vi "parseCCDData.vi"(8 "error in (no error)":errorcluster, 11 "results-JSON string":string) -> (0 "error out":errorcluster, 3 "Array":dbl[][][][](array[numeric]))   [LabVIEW 2023, in "CCD.lvclass"]
uses:
  CCD.lvclass
  dbdbfdab-1b16-4349-82fb-0439317991f3.vi
  <vilib>/JDP Science/JSONtext/Next JSON Value.vi
  <vilib>/JDP Science/JSONtext/String Subset.vi
  <vilib>/JDP Science/JSONtext/Parsing/Advance past next JSON Value (inlined COPY).vi
  <vilib>/JDP Science/JSONtext/Parsing/Advance past whitespace.vi
  <vilib>/JDP Science/JSONtext/Parsing/Advance past String.vi
  <vilib>/JDP Science/JSONtext/Parsing/Advance past Number.vi
  <vilib>/JDP Science/JSONtext/Parsing/Advance past Line Ending.vi
  <vilib>/JDP Science/JSONtext/Parsing/Parse Full Path or Item Name.vi
  <vilib>/JDP Science/JSONtext/Parsing/Advance past Array.vi
  <vilib>/JDP Science/JSONtext/Parsing/Advance past Object.vi
  <vilib>/JDP Science/JSONtext/support/Error Cluster From Code.vi
  <vilib>/JDP Science/JSONtext/Offset/Find Item Locations by Path.vi
  <vilib>/JDP Science/JSONtext/JSON text to Variant.vi
  <vilib>/JDP Science/JSONtext/LVClass Serializer/JSONtext LVClass Serializer.lvclass
  <vilib>/JDP Science/JSONtext/JSONtext.lvlib
  xyData.ctl
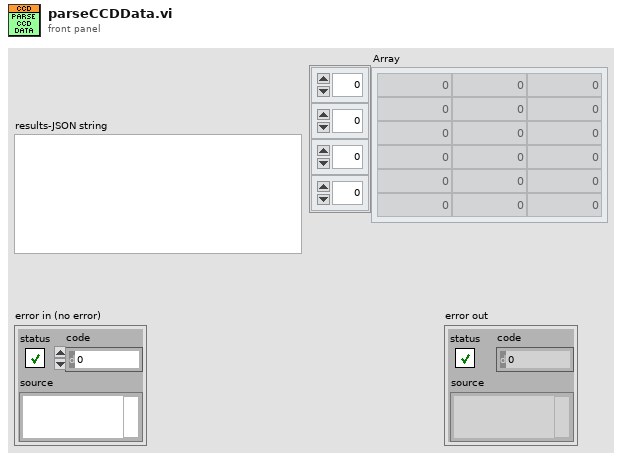
[diagram p1: front panel]
types:
  T1 = typedef "CCD.lvclass/xyData.ctl" = cluster{"xyData":dbl[][]}
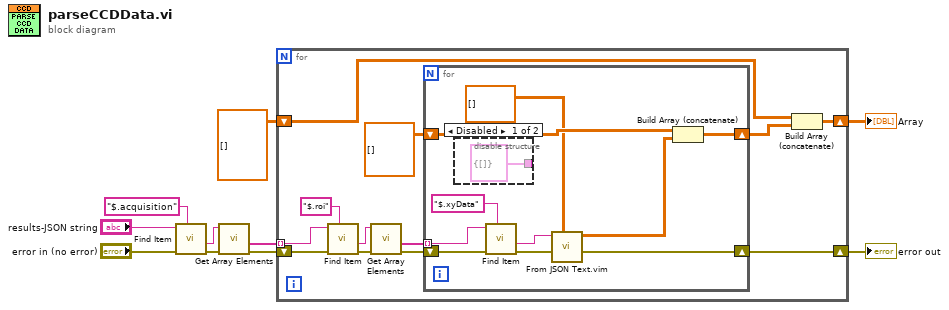
[diagram p0: block diagram]
diagram:
  n1 = call <vilib>:"Find Item.vi"("$Path or Item Name"="$.acquisition", "error in (no error)"="error in (no error)", "JSON"="results-JSON string") -> ("error out"=w7:errorcluster, "<JSON>"=w6:string)  [unwired: 5 in, 2 out]
  n2 = call <vilib>:"Get Array Elements.vi"("error in (no error)"=w7, "JSON"=w6) -> ("error out"=w10:errorcluster, "<JSON>"=w9:string[])  [unwired: 7 in, 1 out]
  n3 = for {
    tunnel: w9 -> [w16] mode=indexing
    shift-right: [w17] -> w5
    shift-left: w10 -> [w19]
    shift-right: [w13] -> w1
    shift-left: dbl[][][][] [] -> [w12]
    n4 = call <vilib>:"Find Item.vi"("$Path or Item Name"="$.roi", "error in (no error)"=w19, "JSON"=w16) -> ("error out"=w21:errorcluster, "<JSON>"=w20:string)  [unwired: 5 in, 2 out]
    n5 = call <vilib>:"Get Array Elements.vi"("error in (no error)"=w21, "JSON"=w20) -> ("error out"=w18:errorcluster, "<JSON>"=w15:string[])  [unwired: 7 in, 1 out]
    n6 = for {
      shift-right: [w28] -> w17
      shift-left: w18 -> [w30]
      tunnel: w15 -> [w31] mode=indexing
      shift-right: [w27] -> w14
      shift-left: dbl[][][] [] -> [w26]
      n7 = disable-structure shown="Disabled" {
        disable-tunnel: [T1 {"xyData"=[]} ("xyData") _] -> _
        frame Disabled {
        }
        frame Enabled {
        }
      }
      n8 = call <vilib>:"Find Item.vi"("$Path or Item Name"="$.xyData", "error in (no error)"=w30, "JSON"=w31) -> ("error out"=w29:errorcluster, "<JSON>"=w25:string)  [unwired: 5 in, 2 out]
      n9 = call "From JSON Text.vim"("Data Type and Default Value"=dbl[][] [], "error in (no error)"=w29, "JSON"=w25) -> ("error out"=w28:errorcluster, "Data out"=w23:dbl[][])  [unwired: 7 in]
      n10 = Build Array (concatenate)(w26, w23) -> (w27:dbl[][][])
    }
    n11 = Build Array (concatenate)(w12, w14) -> (w13:dbl[][][][])
  }
  "error out" <- w5
  "Array" <- w1
